vi "niDTS Comm String Send Command.vi"(0 "Comm String Handle":T1, 5 "Command":string, 7 "Args":string, 11 "error in (no error)":errorcluster) -> (4 "Comm String Handle Out":T1, 6 "Response":string, 15 "error out":errorcluster)   [LabVIEW 2015, in "niDTS CommLib.lvlib"]
doc: "This sends the Command concatenated with the Args over the String Interface.\n\nInputs:\n* Command (Required): This is the command to be sent.\n* Args (Optional): Any arguments to be concatenated with the command.\n\nOutputs:\n* Response: Any data returned from the interface. Note that no data wil be returned if the flag Read Enabled is set to FALSE."
uses:
  niDTS CommLib.lvlib
  Includes/niDTS Comm String INC Handle.ctl
  Objects/String_class/niDTS Comm String.lvclass
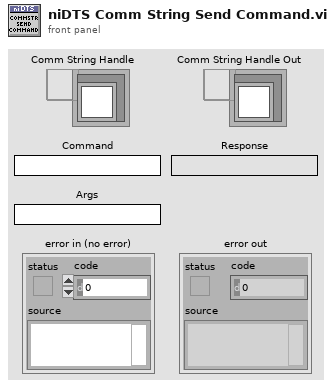
[diagram p1: front panel]
types:
  T1 = typedef "niDTS CommLib.lvlib/niDTS Comm String INC Handle.ctl" = refnum<data-value>
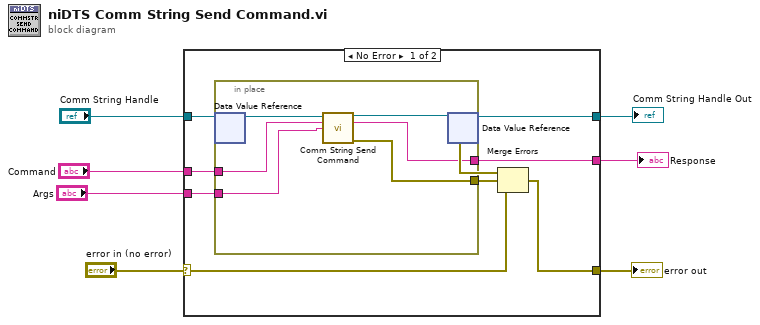
[diagram p0: block diagram]
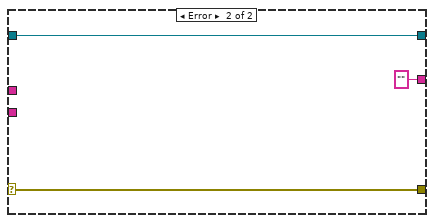
[diagram p2: hidden frame]
diagram:
  n1 = case shown="No Error" "error in (no error)" {
    selector: "error in (no error)" -> [w14 w25]
    tunnel: [w13 w25] -> w7
    tunnel: "Comm String Handle" -> [w16 w24]
    tunnel: [w12 w24] -> w4
    tunnel: "Command" -> [w10 _]
    tunnel: "Args" -> [w9 _]
    tunnel: [w8 "" ("Response")] -> w1
    frame No Error {
      n2 = in-place {
        in-place-border: [w21] -> w11
        in-place-border: w10 -> [w20]
        in-place-border: w9 -> [w19]
        in-place-border: [w17] -> w8
        n3 = in-place-dvr #1(w16) -> (w22:refnum<class "niDTS Comm String.lvclass">)  [unwired: 1 out]
        n4 = call-dynamic "Comm String Send Command.vi"("niDTS Comm String in"=w22, "Command"=w20, "Args"=w19) -> ("niDTS Comm String out"=w18:refnum<class "niDTS Comm String.lvclass">, "Response"=w17:string, "error out"=w21:errorcluster)  [unwired: 10 in]
        n5 = in-place-dvr #1(w18) -> (w12:T1, w15:errorcluster)
      }
      n6 = Merge Errors(w15, w11, w14) -> (w13:errorcluster)
    }
    frame Error {
    }
  }
  "error out" <- w7
  "Comm String Handle Out" <- w4
  "Response" <- w1
